vi "ContourFilledManual2010.vi"   [LabVIEW 2013]
uses:
  ModeType.ctl
  <vilib>/Heliosphere Research LLC/Advanced Plotting Toolkit/api_plotting/ContourFilled_Manual.vi
  <vilib>/Heliosphere Research LLC/Advanced Plotting Toolkit/Advanced Plotting Toolkit.lvlib
types:
  T1 = typedef "ModeType.ctl" = enum16{"Normal", "Expected Failure", "Skipped"}
  T2 = typedef "Advanced Plotting Toolkit.lvlib/PlotID.ctl" = i32
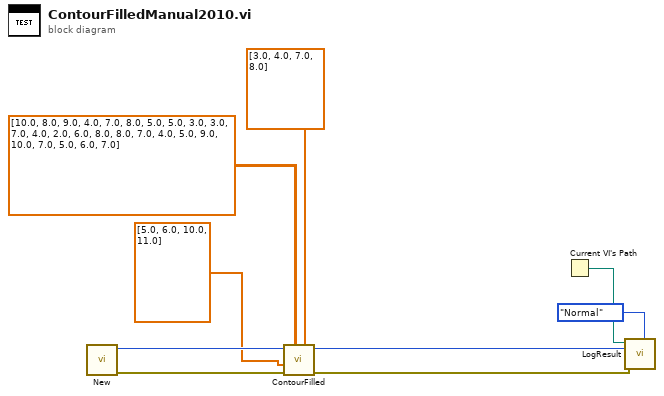
[diagram p0: block diagram]
diagram:
  n1 = call <vilib>:"New.vi"() -> ("error out"=w6:errorcluster, "Plot ID"=w7:T2)  [unwired: 10 in]
  n2 = call-poly <vilib>:"ContourFilled.vi"("Levels"=dbl[] [3.0, 4.0, 7.0, 8.0], "Z Data"=dbl[][] [[10.0, 8.0, 9.0, 4.0, 7.0], [8.0, 5.0, 5.0, 3.0, 3.0], [7.0, 4.0, 2.0, 6.0, 8.0], [8.0, 7.0, 4.0, 5.0, 9.0], [10.0, 7.0, 5.0, 6.0, 7.0]], "error in (no error)"=w6, "Y Coordinates"=dbl[] [5.0, 6.0, 10.0, 11.0] ("X Coordinates"), "Plot ID"=w7) -> ("error out"=w4:errorcluster, "Plot ID Out"=w5:T2)  [unwired: 5 in]
  n3 = Current VI's Path() -> (path=w9:path)
  n4 = call "LogResult.vi"("Mode"=ModeType."Normal", "Test Result"=w4, "Test Artifact"=w5, "VI Path"=w9) -> ()  [unwired: 8 in]
